vi "Sort Circles.vi"(11 "Array 2":T1(array[cluster])) -> (3 "sorted array":T1(array[cluster]))   [LabVIEW 2025]
uses:
  f5cbf16b-9c0e-4588-8f2b-8d026a0dea67.vi
  f5cbf16b-9c0e-4588-8f2b-8d026a0dea67.vi/4611cae3-c7be-41e2-9a5e-ea0ae78a7ced.vi
  f5cbf16b-9c0e-4588-8f2b-8d026a0dea67.vi/4611cae3-c7be-41e2-9a5e-ea0ae78a7ced.vi/19e2e4cb-e3bb-4239-bd5f-680916605f5d.vi
  f5cbf16b-9c0e-4588-8f2b-8d026a0dea67.vi/4611cae3-c7be-41e2-9a5e-ea0ae78a7ced.vi/f72612c1-738a-48a1-9fcf-3db66cb27fb3.vi
  f5cbf16b-9c0e-4588-8f2b-8d026a0dea67.vi/4611cae3-c7be-41e2-9a5e-ea0ae78a7ced.vi/45406051-8994-464b-8b47-ac12a8cbadfa.vi
  f5cbf16b-9c0e-4588-8f2b-8d026a0dea67.vi/4611cae3-c7be-41e2-9a5e-ea0ae78a7ced.vi/dd886480-778c-48b1-8e4a-d6890e1a60dd.vi
  f5cbf16b-9c0e-4588-8f2b-8d026a0dea67.vi/4611cae3-c7be-41e2-9a5e-ea0ae78a7ced.vi/2e6e140f-e361-4312-a09e-e37273ac7fd1.vi
  f5cbf16b-9c0e-4588-8f2b-8d026a0dea67.vi/4611cae3-c7be-41e2-9a5e-ea0ae78a7ced.vi/3589548e-4c68-4568-af05-72ab28470577.vi
  f5cbf16b-9c0e-4588-8f2b-8d026a0dea67.vi/4611cae3-c7be-41e2-9a5e-ea0ae78a7ced.vi/cf64d4f5-91bd-4749-9577-68c6ded0155b.vi
  f5cbf16b-9c0e-4588-8f2b-8d026a0dea67.vi/4611cae3-c7be-41e2-9a5e-ea0ae78a7ced.vi/6f6fefe9-f25b-4595-b26f-75715299a794.vi
  f5cbf16b-9c0e-4588-8f2b-8d026a0dea67.vi/4611cae3-c7be-41e2-9a5e-ea0ae78a7ced.vi/c74ffb76-1048-4639-9a95-b6de96ba7014.vi
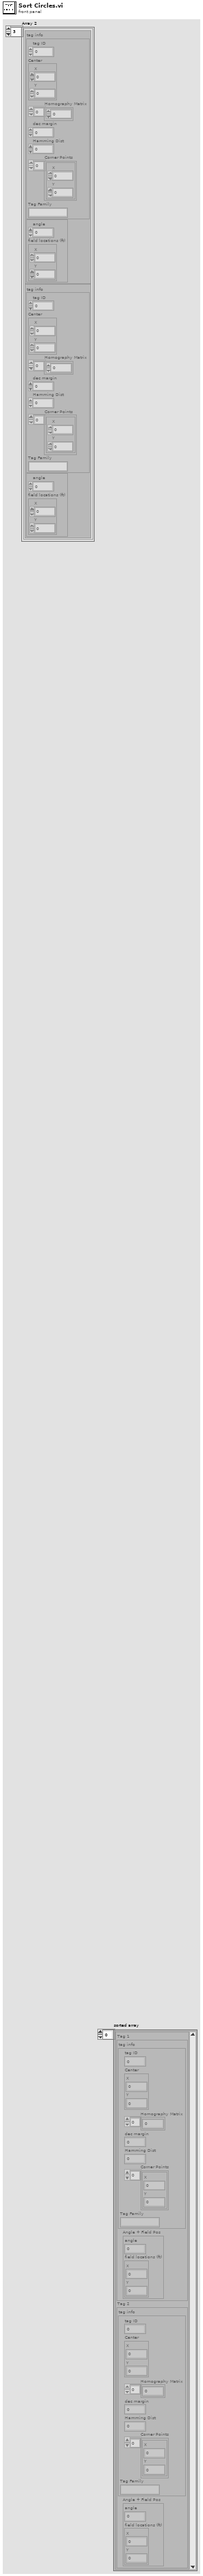
[diagram p1: front panel]
types:
  T1 = cluster{"Tag 1":cluster{"tag info":cluster{"tag ID":i32, "Center":cluster{"X":dbl, "Y":dbl}, "Homography Matrix":dbl[], "dec margin":dbl, "Hamming Dist":i32, "Corner Points":cluster{"X":dbl, "Y":dbl}[], "Tag Family":string}, "Angle + Field Pos":cluster{"angle":dbl, "field locations (ft)":cluster{"X":dbl, "Y":dbl}}}, "Tag 2":cluster{"tag info":cluster{"tag ID":i32, "Center":cluster{"X":dbl, "Y":dbl}, "Homography Matrix":dbl[], "dec margin":dbl, "Hamming Dist":i32, "Corner Points":cluster{"X":dbl, "Y":dbl}[], "Tag Family":string}, "Angle + Field Pos":cluster{"angle":dbl, "field locations (ft)":cluster{"X":dbl, "Y":dbl}}}}[]
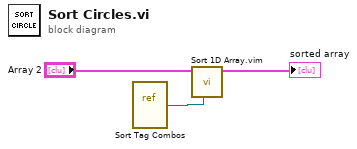
[diagram p0: block diagram]
diagram:
  n1 = vi-ref "Sort Tag Combos.vi"() -> (w2:refnum<vi>)
  n2 = call "Sort 1D Array.vim"("less function (built-in <)"=w2, "unsorted array"="Array 2") -> ("sorted array"=→"sorted array":T1)  [unwired: 9 in]
